vi "Configure Control - Control Limits.vi"(8 "error in (no error)":errorcluster, 10 "control in":refnum<vi>, 11 "Has Control Limits in":refnum<class "Has Control Limits.lvclass">) -> (0 "error out":errorcluster, 2 "control out":refnum<vi>, 3 "Has Control Limits out":refnum<class "Has Control Limits.lvclass">)   [LabVIEW 2020, in "PV Access.lvlib" / "PV Data.lvlib" / "Has Control Limits.lvclass"]
uses:
  Has Control Limits.lvclass
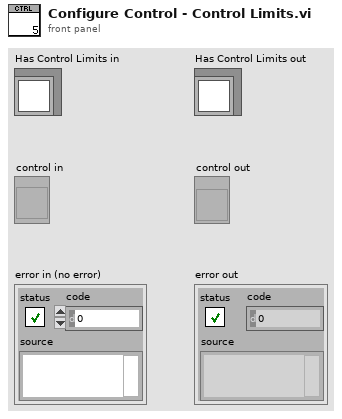
[diagram p1: front panel]
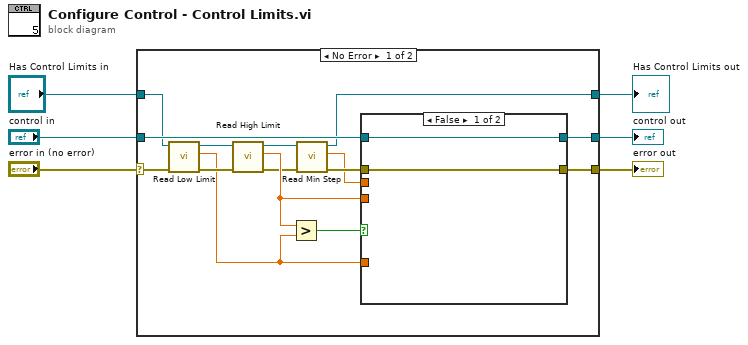
[diagram p0: block diagram]
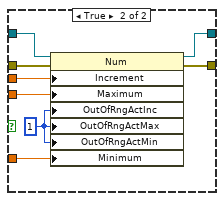
[diagram p2: hidden frame]
diagram:
  n1 = case shown="No Error" "error in (no error)" {
    selector: "error in (no error)" -> [w17 w33]
    tunnel: [w21 w33] -> w2
    tunnel: [w19 w32] -> w1
    tunnel: [w9 w34] -> w3
    tunnel: "Has Control Limits in" -> [w16 w34]
    tunnel: "control in" -> [w18 w32]
    frame No Error {
      n2 = call-dynamic "Read Low Limit.vi"("error in"=w17, "Has Control Limits in"=w16) -> ("error out"=w13:errorcluster, "low limit"=w7:dbl, "Has Control Limits out"=w10:refnum<class "Has Control Limits.lvclass">)  [unwired: 7 in]
      n3 = call-dynamic "Read High Limit.vi"("error in"=w13, "Has Control Limits in"=w10) -> ("error out"=w12:errorcluster, "high limit"=w15:dbl, "Has Control Limits out"=w11:refnum<class "Has Control Limits.lvclass">)  [unwired: 7 in]
      n4 = Greater?(x=w15, y=w7) -> (0:w20:bool)
      n5 = call-dynamic "Read Min Step.vi"("error in"=w12, "Has Control Limits in"=w11) -> ("error out"=w14:errorcluster, "min step"=w8:dbl, "Has Control Limits out"=w9:refnum<class "Has Control Limits.lvclass">)  [unwired: 7 in]
      n6 = case shown="False" w20 {
        tunnel: [w23 w31] -> w21
        tunnel: w18 -> [w22 w30]
        tunnel: w8 -> [_ w29]
        tunnel: w15 -> [_ w28]
        tunnel: w7 -> [_ w24]
        tunnel: w14 -> [w23 w27]
        tunnel: [w22 w25] -> w19
        frame False {
        }
        frame True {
          w26 = u8 1 ("Response to Value Outside Limits:Minimum")
          n7 = property on="Property Node" class="Num"(reference=w30, error in=w27, "Increment"=w29, "Maximum"=w28, "OutOfRngActInc"=w26, "OutOfRngActMax"=w26, "OutOfRngActMin"=w26, "Minimum"=w24) -> (reference out=w25:refnum<vi>, error out=w31:errorcluster)
        }
      }
    }
    frame Error {
    }
  }
  "error out" <- w2
  "Has Control Limits out" <- w3
  "control out" <- w1
